vi "Counter.to.nm.vi"(11 "Mono in":T1) -> (3 "Mono out":T1)   [LabVIEW 2022 SP3]
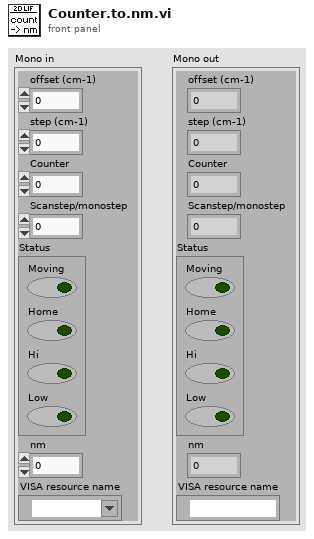
[diagram p1: front panel]
types:
  T1 = cluster{"offset (cm-1)":dbl, "step (cm-1)":dbl, "Counter":dbl, "Scanstep/monostep":i32, "Status":cluster{"Moving":bool, "Home":bool, "Hi":bool, "Low":bool}, "nm":dbl, "VISA resource name":refnum<visa-resource-name>}
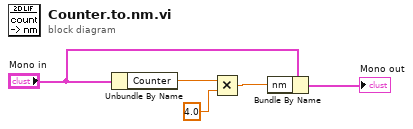
[diagram p0: block diagram]
diagram:
  n1 = Unbundle By Name("Mono in") -> ("Counter"=w1:dbl)
  n2 = Multiply(x=w1, y=4.0) -> (x*y=w4:dbl)
  n3 = Bundle By Name(cluster="Mono in", "nm"=w4) -> (→"Mono out":T1)
